vi "Translator.vi"(0 "Input":variant, 11 "error in (no error)":errorcluster) -> (4 "Output":variant, 15 "error out":errorcluster)   [LabVIEW 2014, in "Complex Numbers.lvlib"]
doc: "An example of how to create the Translator to convert the LabVIEW VIs to Arduino C code."
uses:
  Complex Numbers.lvlib
panel:
  out "Outputs":string[](array[string])
  out "Inputs":string[](array[string])
  out "Output Datatypes":string[](array[string])
  out "Input Datatypes":string[](array[string])
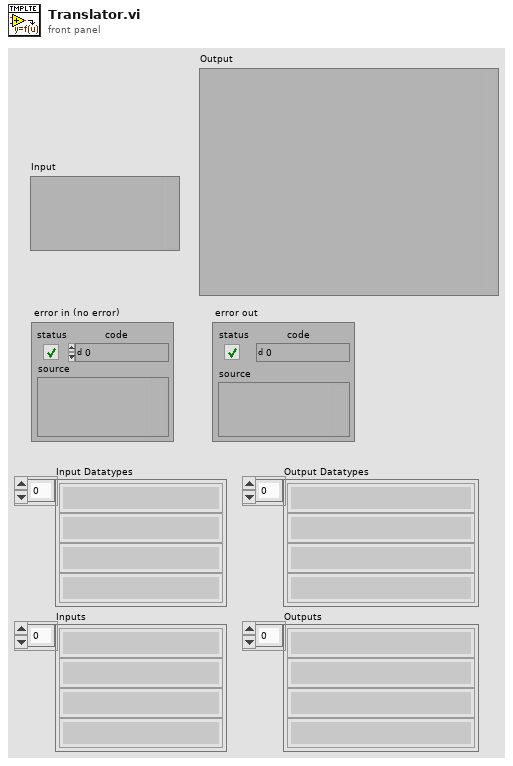
[diagram p1: front panel]
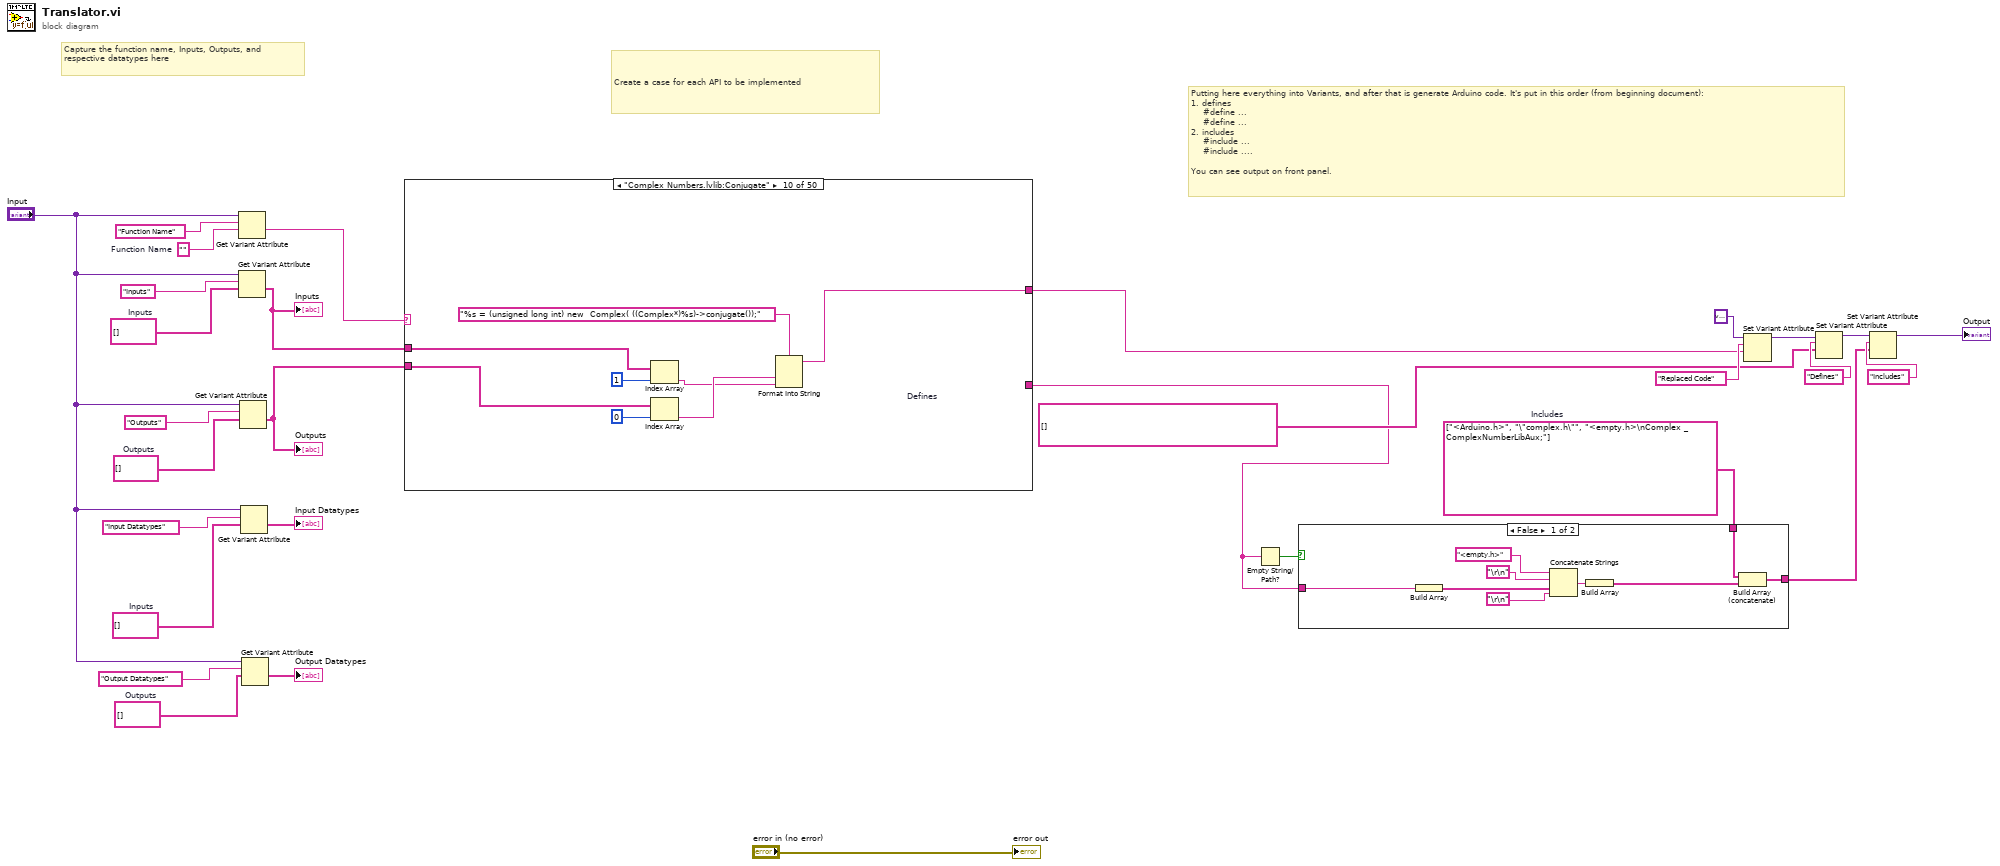
[diagram p0: block diagram]
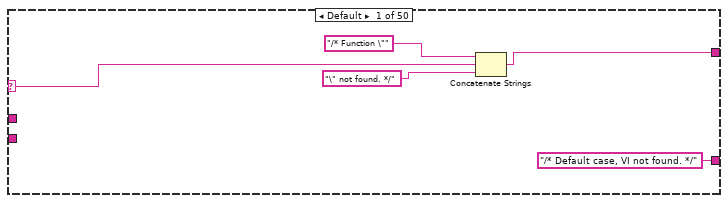
[diagram p3: hidden frame]
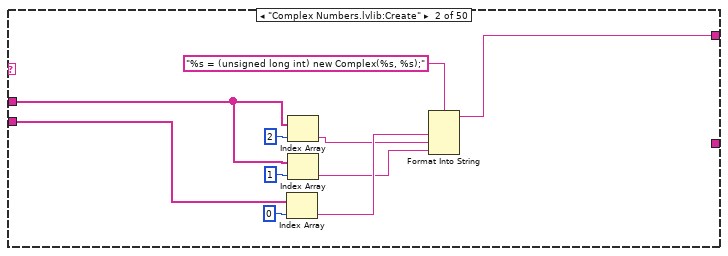
[diagram p4: hidden frame]
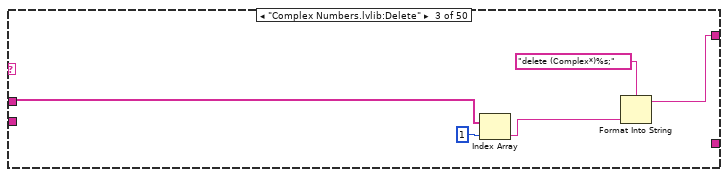
[diagram p5: hidden frame]
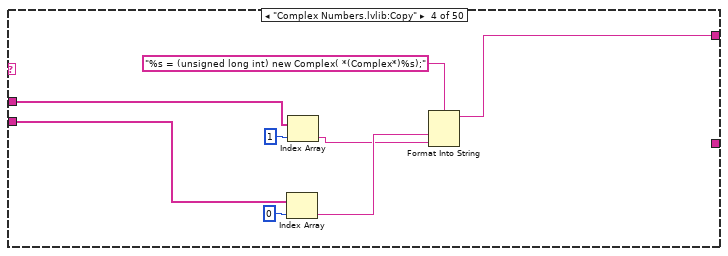
[diagram p6: hidden frame]
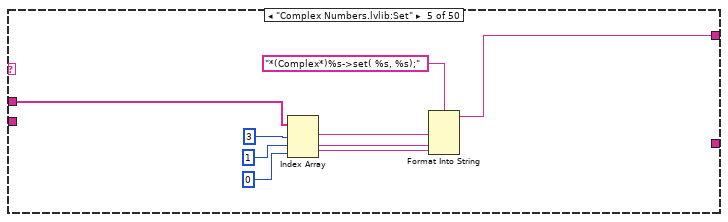
[diagram p7: hidden frame]
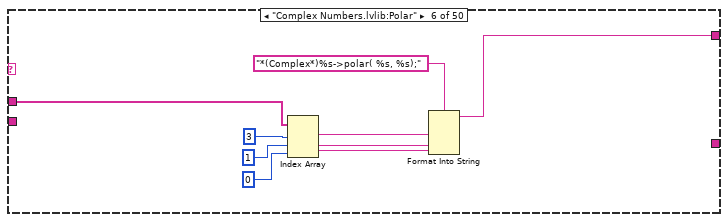
[diagram p8: hidden frame]
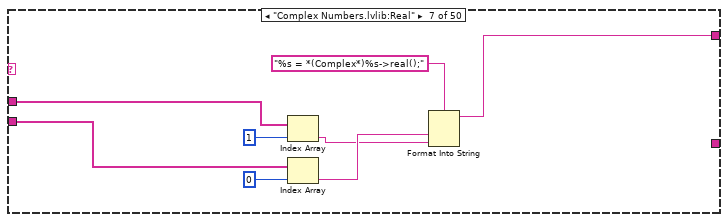
[diagram p9: hidden frame]
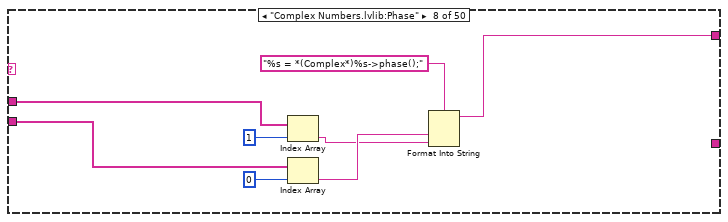
[diagram p10: hidden frame]
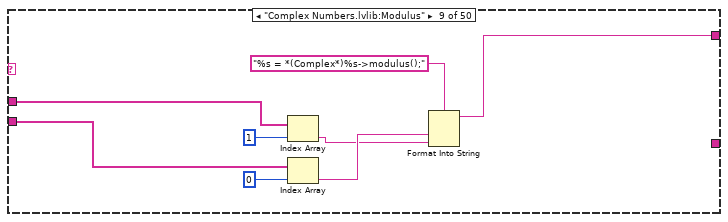
[diagram p11: hidden frame]
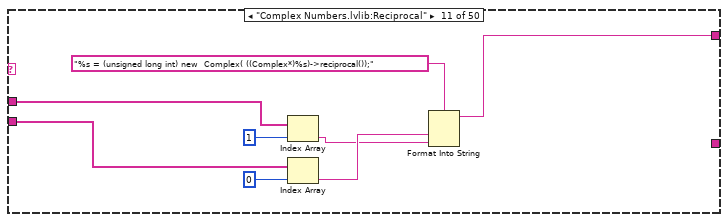
[diagram p12: hidden frame]
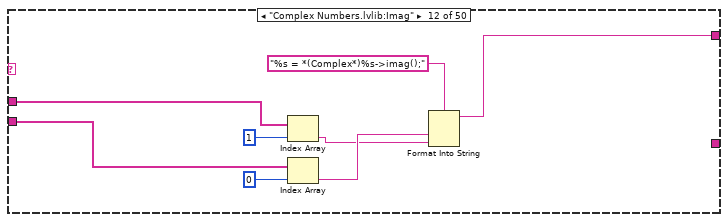
[diagram p13: hidden frame]
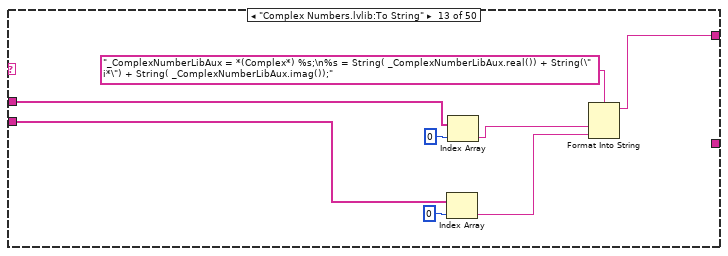
[diagram p14: hidden frame]
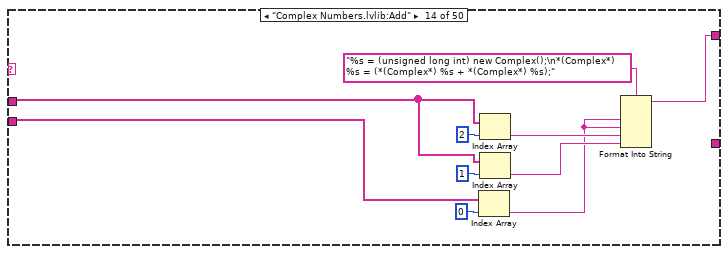
[diagram p15: hidden frame]
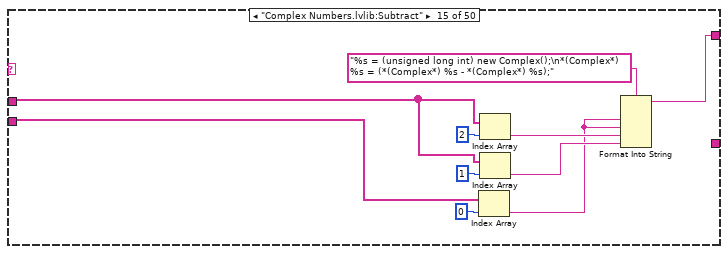
[diagram p16: hidden frame]
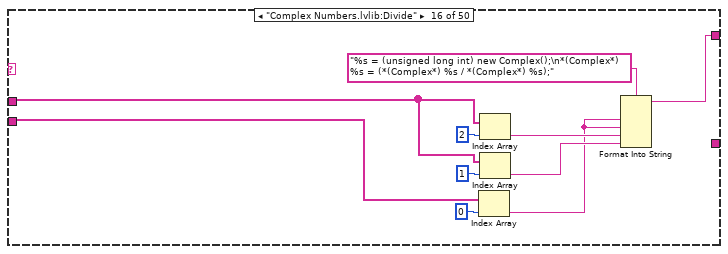
[diagram p17: hidden frame]
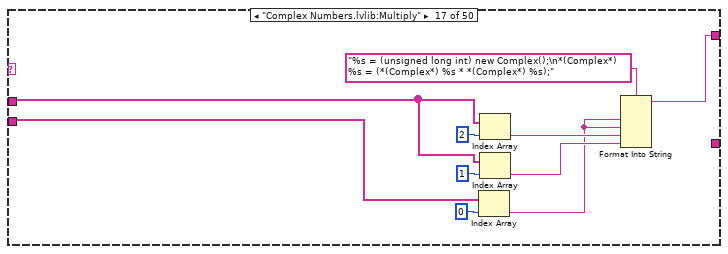
[diagram p18: hidden frame]
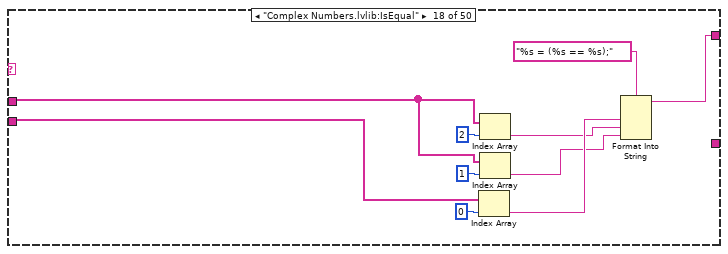
[diagram p19: hidden frame]
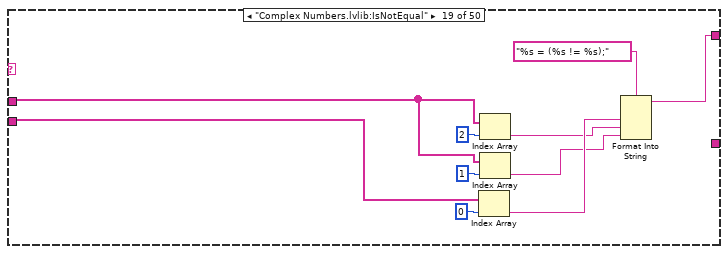
[diagram p20: hidden frame]
diagram:
  w4 = string[] []  # Defines
  w19 = string[] []  # Outputs
  w20 = string[] []  # Inputs
  w1 = string[] ["<Arduino.h>", "\"complex.h\"", "<empty.h>\nComplex _ComplexNumberLibAux;"]  # Includes
  w26 = string[] []  # Outputs
  w27 = string[] []  # Inputs
  w28 = ""  # Function Name
  # "Capture the function name, Inputs, Outputs, and respective datatypes here"
  # "Putting here everything into Variants, and after that is generate Arduino code. It's put in this order (from beginning document):\n1. defines\n    #define ...\n    #define ...\n2. includes\n    #include ...\n    #include ....\n\nYou can see output on front panel."
  # "Create a case for each API to be implemented"
  n1 = Get Variant Attribute(Variant="Input", name="Function Name", default value (empty Variant)=w28) -> (value=w10:string)  [unwired: 1 in, 3 out]
  n2 = Get Variant Attribute(Variant="Input", name="Inputs", default value (empty Variant)=w27) -> (value=w9:string[])  [unwired: 1 in, 3 out]
  "Inputs" <- w9
  n3 = Get Variant Attribute(Variant="Input", name="Outputs", default value (empty Variant)=w26) -> (value=w8:string[])  [unwired: 1 in, 3 out]
  "Outputs" <- w8
  n4 = Get Variant Attribute(Variant="Input", name="Input Datatypes", default value (empty Variant)=w20) -> (value=→"Input Datatypes":string[])  [unwired: 1 in, 3 out]
  n5 = Get Variant Attribute(Variant="Input", name="Output Datatypes", default value (empty Variant)=w19) -> (value=→"Output Datatypes":string[])  [unwired: 1 in, 3 out]
  n6 = case shown="\"Complex Numbers.lvlib:Conjugate\"" w10 {
    selector: w10 -> [w33 _ _ _ _ _ _ _ _ _ _ _ _ _ _ _ _ _ _ _ _ _ _ _ _ _ _ _ _ _ _ _ _ _ _ _ _ _ _ _ _ _ _ _ _ _ _ _ _ _]
    tunnel: w9 -> [_ w38 w48 w52 w64 w73 w80 w88 w96 w104 w112 w120 w126 w136 w146 w156 w166 w177 w187 w196 w204 w210 w222 w230 w238 w244 w256 w264 w272 w280 w288 w296 w304 w312 w320 w328 w336 w344 w352 w360 w368 w376 w384 w392 w400 w408 w416 w424 w432 w440]
    tunnel: w8 -> [_ w42 _ w55 _ _ w79 w87 w95 w103 w111 w119 w129 w138 w148 w158 w168 w179 w189 w197 w205 w215 w223 w231 w239 w249 w257 w265 w273 w281 w289 w297 w305 w313 w321 w329 w337 w345 w353 w361 w369 w377 w385 w393 w401 w409 w417 w425 w433 w441]
    tunnel: [w31 w41 w47 w54 w66 w75 w83 w91 w99 w107 w115 w123 w128 w134 w144 w154 w164 w176 w186 w195 w203 w214 w221 w229 w237 w248 w255 w263 w271 w279 w287 w295 w303 w311 w319 w327 w335 w343 w351 w359 w367 w375 w383 w391 w399 w407 w415 w423 w431 w439] -> w7
    tunnel: ["/* Default case, VI not found. */" ("name") _ _ _ _ _ _ _ _ _ _ _ _ _ _ _ _ _ _ _ _ _ _ _ _ _ _ _ _ _ _ _ _ _ _ _ _ _ _ _ _ _ _ _ _ _ _ _ _ _] -> w3
    frame Default {
      n7 = Concatenate Strings("/* Function \"" ("string"), w33, "\" not found. */" ("string")) -> (w31:string)
    }
    frame "Complex Numbers.lvlib:Create" {
      n8 = Index Array(array=w42, index=0) -> (element=w44:string)
      n9 = Index Array(array=w38, index=2) -> (element=w37:string)
      n10 = Index Array(array=w38, index=1) -> (element=w36:string)
      n11 = Format Into String(format string="%s = (unsigned long int) new Complex(%s, %s);", w44, w37, w36) -> (resulting string=w41:string)  [unwired: 2 in, 1 out]
    }
    frame "Complex Numbers.lvlib:Delete" {
      n12 = Index Array(array=w48, index=1) -> (element=w46:string)
      n13 = Format Into String(format string="delete (Complex*)%s;", w46) -> (resulting string=w47:string)  [unwired: 2 in, 1 out]
    }
    frame "Complex Numbers.lvlib:Copy" {
      n14 = Index Array(array=w55, index=0) -> (element=w57:string)
      n15 = Index Array(array=w52, index=1) -> (element=w51:string)
      n16 = Format Into String(format string="%s = (unsigned long int) new Complex( *(Complex*)%s);", w57, w51) -> (resulting string=w54:string)  [unwired: 2 in, 1 out]
    }
    frame "Complex Numbers.lvlib:Set" {
      n17 = Index Array(array=w64, index #1=3 ("index"), index #2=1 ("index"), index #3=0 ("index")) -> (element #1=w61:string, element #2=w60:string, element #3=w59:string)
      n18 = Format Into String(format string="*(Complex*)%s->set( %s, %s);", w61, w60, w59) -> (resulting string=w66:string)  [unwired: 2 in, 1 out]
    }
    frame "Complex Numbers.lvlib:Polar" {
      n19 = Index Array(array=w73, index #1=3 ("index"), index #2=1 ("index"), index #3=0 ("index")) -> (element #1=w70:string, element #2=w69:string, element #3=w68:string)
      n20 = Format Into String(format string="*(Complex*)%s->polar( %s, %s);", w70, w69, w68) -> (resulting string=w75:string)  [unwired: 2 in, 1 out]
    }
    frame "Complex Numbers.lvlib:Real" {
      n21 = Index Array(array=w80, index=1) -> (element=w77:string)
      n22 = Index Array(array=w79, index=0) -> (element=w78:string)
      n23 = Format Into String(format string="%s = *(Complex*)%s->real();", w78, w77) -> (resulting string=w83:string)  [unwired: 2 in, 1 out]
    }
    frame "Complex Numbers.lvlib:Phase" {
      n24 = Index Array(array=w88, index=1) -> (element=w85:string)
      n25 = Index Array(array=w87, index=0) -> (element=w86:string)
      n26 = Format Into String(format string="%s = *(Complex*)%s->phase();", w86, w85) -> (resulting string=w91:string)  [unwired: 2 in, 1 out]
    }
    frame "Complex Numbers.lvlib:Modulus" {
      n27 = Index Array(array=w96, index=1) -> (element=w93:string)
      n28 = Index Array(array=w95, index=0) -> (element=w94:string)
      n29 = Format Into String(format string="%s = *(Complex*)%s->modulus();", w94, w93) -> (resulting string=w99:string)  [unwired: 2 in, 1 out]
    }
    frame "Complex Numbers.lvlib:Conjugate" {
      n30 = Index Array(array=w104, index=1) -> (element=w101:string)
      n31 = Index Array(array=w103, index=0) -> (element=w102:string)
      n32 = Format Into String(format string="%s = (unsigned long int) new  Complex( ((Complex*)%s)->conjugate());", w102, w101) -> (resulting string=w107:string)  [unwired: 2 in, 1 out]
    }
    frame "Complex Numbers.lvlib:Reciprocal" {
      n33 = Index Array(array=w112, index=1) -> (element=w109:string)
      n34 = Index Array(array=w111, index=0) -> (element=w110:string)
      n35 = Format Into String(format string="%s = (unsigned long int) new  Complex( ((Complex*)%s)->reciprocal());", w110, w109) -> (resulting string=w115:string)  [unwired: 2 in, 1 out]
    }
    frame "Complex Numbers.lvlib:Imag" {
      n36 = Index Array(array=w120, index=1) -> (element=w117:string)
      n37 = Index Array(array=w119, index=0) -> (element=w118:string)
      n38 = Format Into String(format string="%s = *(Complex*)%s->imag();", w118, w117) -> (resulting string=w123:string)  [unwired: 2 in, 1 out]
    }
    frame "Complex Numbers.lvlib:To String" {
      n39 = Index Array(array=w129, index=0) -> (element=w131:string)
      n40 = Index Array(array=w126, index=0) -> (element=w125:string)
      n41 = Format Into String(format string="_ComplexNumberLibAux = *(Complex*) %s;\n%s = String( _ComplexNumberLibAux.real()) + String(\" i*\") + String( _ComplexNumberLibAux.imag());", w125, w131) -> (resulting string=w128:string)  [unwired: 2 in, 1 out]
    }
    frame "Complex Numbers.lvlib:Add" {
      n42 = Index Array(array=w138, index=0) -> (element=w133:string)
      n43 = Index Array(array=w136, index=2) -> (element=w142:string)
      n44 = Index Array(array=w136, index=1) -> (element=w135:string)
      n45 = Format Into String(format string="%s = (unsigned long int) new Complex();\n*(Complex*) %s = (*(Complex*) %s + *(Complex*) %s);", w133, w133, w142, w135) -> (resulting string=w134:string)  [unwired: 2 in, 1 out]
    }
    frame "Complex Numbers.lvlib:Subtract" {
      n46 = Index Array(array=w148, index=0) -> (element=w143:string)
      n47 = Index Array(array=w146, index=2) -> (element=w152:string)
      n48 = Index Array(array=w146, index=1) -> (element=w145:string)
      n49 = Format Into String(format string="%s = (unsigned long int) new Complex();\n*(Complex*) %s = (*(Complex*) %s - *(Complex*) %s);", w143, w143, w152, w145) -> (resulting string=w144:string)  [unwired: 2 in, 1 out]
    }
    frame "Complex Numbers.lvlib:Divide" {
      n50 = Index Array(array=w158, index=0) -> (element=w153:string)
      n51 = Index Array(array=w156, index=2) -> (element=w162:string)
      n52 = Index Array(array=w156, index=1) -> (element=w155:string)
      n53 = Format Into String(format string="%s = (unsigned long int) new Complex();\n*(Complex*) %s = (*(Complex*) %s / *(Complex*) %s);", w153, w153, w162, w155) -> (resulting string=w154:string)  [unwired: 2 in, 1 out]
    }
    frame "Complex Numbers.lvlib:Multiply" {
      n54 = Index Array(array=w168, index=0) -> (element=w163:string)
      n55 = Index Array(array=w166, index=2) -> (element=w172:string)
      n56 = Index Array(array=w166, index=1) -> (element=w165:string)
      n57 = Format Into String(format string="%s = (unsigned long int) new Complex();\n*(Complex*) %s = (*(Complex*) %s * *(Complex*) %s);", w163, w163, w172, w165) -> (resulting string=w164:string)  [unwired: 2 in, 1 out]
    }
    frame "Complex Numbers.lvlib:IsEqual" {
      n58 = Index Array(array=w179, index=0) -> (element=w175:string)
      n59 = Index Array(array=w177, index=2) -> (element=w174:string)
      n60 = Index Array(array=w177, index=1) -> (element=w173:string)
      n61 = Format Into String(format string="%s = (%s == %s);", w175, w174, w173) -> (resulting string=w176:string)  [unwired: 2 in, 1 out]
    }
    frame "Complex Numbers.lvlib:IsNotEqual" {
      n62 = Index Array(array=w189, index=0) -> (element=w185:string)
      n63 = Index Array(array=w187, index=2) -> (element=w184:string)
      n64 = Index Array(array=w187, index=1) -> (element=w183:string)
      n65 = Format Into String(format string="%s = (%s != %s);", w185, w184, w183) -> (resulting string=w186:string)  [unwired: 2 in, 1 out]
    }
    frame "Complex Numbers.lvlib:Sqr" {
      n66 = Index Array(array=w197, index=0) -> (element=w194:string)
      n67 = Index Array(array=w196, index=1) -> (element=w193:string)
      n68 = Format Into String(format string="%s = (unsigned long int) new Complex( ((Complex*)%s)->c_sqr());", w194, w193) -> (resulting string=w195:string)  [unwired: 2 in, 1 out]
    }
    frame "Complex Numbers.lvlib:Sqrt" {
      n69 = Index Array(array=w205, index=0) -> (element=w202:string)
      n70 = Index Array(array=w204, index=1) -> (element=w201:string)
      n71 = Format Into String(format string="%s = (unsigned long int) new Complex( ((Complex*)%s)->c_sqrt());", w202, w201) -> (resulting string=w203:string)  [unwired: 2 in, 1 out]
    }
    frame "Complex Numbers.lvlib:Pow" {
      n72 = Index Array(array=w215, index=0) -> (element=w213:string)
      n73 = Index Array(array=w210, index=2) -> (element=w212:string)
      n74 = Index Array(array=w210, index=1) -> (element=w209:string)
      n75 = Format Into String(format string="%s = (unsigned long int) new Complex( ((Complex*)%s)->c_pow( *(Complex*)%s));", w213, w212, w209) -> (resulting string=w214:string)  [unwired: 2 in, 1 out]
    }
    frame "Complex Numbers.lvlib:Exp" {
      n76 = Index Array(array=w223, index=0) -> (element=w220:string)
      n77 = Index Array(array=w222, index=1) -> (element=w219:string)
      n78 = Format Into String(format string="%s = (unsigned long int) new Complex( ((Complex*)%s)->c_exp());", w220, w219) -> (resulting string=w221:string)  [unwired: 2 in, 1 out]
    }
    frame "Complex Numbers.lvlib:Log" {
      n79 = Index Array(array=w231, index=0) -> (element=w228:string)
      n80 = Index Array(array=w230, index=1) -> (element=w227:string)
      n81 = Format Into String(format string="%s = (unsigned long int) new Complex( ((Complex*)%s)->c_log());", w228, w227) -> (resulting string=w229:string)  [unwired: 2 in, 1 out]
    }
    frame "Complex Numbers.lvlib:Log10" {
      n82 = Index Array(array=w239, index=0) -> (element=w236:string)
      n83 = Index Array(array=w238, index=1) -> (element=w235:string)
      n84 = Format Into String(format string="%s = (unsigned long int) new Complex( ((Complex*)%s)->c_log10());", w236, w235) -> (resulting string=w237:string)  [unwired: 2 in, 1 out]
    }
    frame "Complex Numbers.lvlib:LogN" {
      n85 = Index Array(array=w249, index=0) -> (element=w247:string)
      n86 = Index Array(array=w244, index=2) -> (element=w246:string)
      n87 = Index Array(array=w244, index=1) -> (element=w243:string)
      n88 = Format Into String(format string="%s = (unsigned long int) new Complex( ((Complex*)%s)->c_logn( *(Complex*)%s));", w247, w246, w243) -> (resulting string=w248:string)  [unwired: 2 in, 1 out]
    }
    frame "Complex Numbers.lvlib:Sin" {
      n89 = Index Array(array=w257, index=0) -> (element=w254:string)
      n90 = Index Array(array=w256, index=1) -> (element=w253:string)
      n91 = Format Into String(format string="%s = (unsigned long int) new Complex( ((Complex*)%s)->c_sin());", w254, w253) -> (resulting string=w255:string)  [unwired: 2 in, 1 out]
    }
    frame "Complex Numbers.lvlib:Cos" {
      n92 = Index Array(array=w265, index=0) -> (element=w262:string)
      n93 = Index Array(array=w264, index=1) -> (element=w261:string)
      n94 = Format Into String(format string="%s = (unsigned long int) new Complex( ((Complex*)%s)->c_cos());", w262, w261) -> (resulting string=w263:string)  [unwired: 2 in, 1 out]
    }
    frame "Complex Numbers.lvlib:Tan" {
      n95 = Index Array(array=w273, index=0) -> (element=w270:string)
      n96 = Index Array(array=w272, index=1) -> (element=w269:string)
      n97 = Format Into String(format string="%s = (unsigned long int) new Complex( ((Complex*)%s)->c_tan());", w270, w269) -> (resulting string=w271:string)  [unwired: 2 in, 1 out]
    }
    frame "Complex Numbers.lvlib:Cot" {
      n98 = Index Array(array=w281, index=0) -> (element=w278:string)
      n99 = Index Array(array=w280, index=1) -> (element=w277:string)
      n100 = Format Into String(format string="%s = (unsigned long int) new Complex( ((Complex*)%s)->c_cot());", w278, w277) -> (resulting string=w279:string)  [unwired: 2 in, 1 out]
    }
    frame "Complex Numbers.lvlib:Asin" {
      n101 = Index Array(array=w289, index=0) -> (element=w286:string)
      n102 = Index Array(array=w288, index=1) -> (element=w285:string)
      n103 = Format Into String(format string="%s = (unsigned long int) new Complex( ((Complex*)%s)->c_asin());", w286, w285) -> (resulting string=w287:string)  [unwired: 2 in, 1 out]
    }
    frame "Complex Numbers.lvlib:Acos" {
      n104 = Index Array(array=w297, index=0) -> (element=w294:string)
      n105 = Index Array(array=w296, index=1) -> (element=w293:string)
      n106 = Format Into String(format string="%s = (unsigned long int) new Complex( ((Complex*)%s)->c_acos());", w294, w293) -> (resulting string=w295:string)  [unwired: 2 in, 1 out]
    }
    frame "Complex Numbers.lvlib:Atan" {
      n107 = Index Array(array=w305, index=0) -> (element=w302:string)
      n108 = Index Array(array=w304, index=1) -> (element=w301:string)
      n109 = Format Into String(format string="%s = (unsigned long int) new Complex( ((Complex*)%s)->c_atan());", w302, w301) -> (resulting string=w303:string)  [unwired: 2 in, 1 out]
    }
    frame "Complex Numbers.lvlib:Acot" {
      n110 = Index Array(array=w313, index=0) -> (element=w310:string)
      n111 = Index Array(array=w312, index=1) -> (element=w309:string)
      n112 = Format Into String(format string="%s = (unsigned long int) new Complex( ((Complex*)%s)->c_acot());", w310, w309) -> (resulting string=w311:string)  [unwired: 2 in, 1 out]
    }
    frame "Complex Numbers.lvlib:Csc" {
      n113 = Index Array(array=w321, index=0) -> (element=w318:string)
      n114 = Index Array(array=w320, index=1) -> (element=w317:string)
      n115 = Format Into String(format string="%s = (unsigned long int) new Complex( ((Complex*)%s)->c_csc());", w318, w317) -> (resulting string=w319:string)  [unwired: 2 in, 1 out]
    }
    frame "Complex Numbers.lvlib:Sec" {
      n116 = Index Array(array=w329, index=0) -> (element=w326:string)
      n117 = Index Array(array=w328, index=1) -> (element=w325:string)
      n118 = Format Into String(format string="%s = (unsigned long int) new Complex( ((Complex*)%s)->c_sec());", w326, w325) -> (resulting string=w327:string)  [unwired: 2 in, 1 out]
    }
    frame "Complex Numbers.lvlib:Acsc" {
      n119 = Index Array(array=w337, index=0) -> (element=w334:string)
      n120 = Index Array(array=w336, index=1) -> (element=w333:string)
      n121 = Format Into String(format string="%s = (unsigned long int) new Complex( ((Complex*)%s)->c_acsc());", w334, w333) -> (resulting string=w335:string)  [unwired: 2 in, 1 out]
    }
    frame "Complex Numbers.lvlib:Asec" {
      n122 = Index Array(array=w345, index=0) -> (element=w342:string)
      n123 = Index Array(array=w344, index=1) -> (element=w341:string)
      n124 = Format Into String(format string="%s = (unsigned long int) new Complex( ((Complex*)%s)->c_asec());", w342, w341) -> (resulting string=w343:string)  [unwired: 2 in, 1 out]
    }
    frame "Complex Numbers.lvlib:Sinh" {
      n125 = Index Array(array=w353, index=0) -> (element=w350:string)
      n126 = Index Array(array=w352, index=1) -> (element=w349:string)
      n127 = Format Into String(format string="%s = (unsigned long int) new Complex( ((Complex*)%s)->c_sinh());", w350, w349) -> (resulting string=w351:string)  [unwired: 2 in, 1 out]
    }
    frame "Complex Numbers.lvlib:Cosh" {
      n128 = Index Array(array=w361, index=0) -> (element=w358:string)
      n129 = Index Array(array=w360, index=1) -> (element=w357:string)
      n130 = Format Into String(format string="%s = (unsigned long int) new Complex( ((Complex*)%s)->c_cosh());", w358, w357) -> (resulting string=w359:string)  [unwired: 2 in, 1 out]
    }
    frame "Complex Numbers.lvlib:Tanh" {
      n131 = Index Array(array=w369, index=0) -> (element=w366:string)
      n132 = Index Array(array=w368, index=1) -> (element=w365:string)
      n133 = Format Into String(format string="%s = (unsigned long int) new Complex( ((Complex*)%s)->c_tanh());", w366, w365) -> (resulting string=w367:string)  [unwired: 2 in, 1 out]
    }
    frame "Complex Numbers.lvlib:Asinh" {
      n134 = Index Array(array=w377, index=0) -> (element=w374:string)
      n135 = Index Array(array=w376, index=1) -> (element=w373:string)
      n136 = Format Into String(format string="%s = (unsigned long int) new Complex( ((Complex*)%s)->c_asinh());", w374, w373) -> (resulting string=w375:string)  [unwired: 2 in, 1 out]
    }
    frame "Complex Numbers.lvlib:Acosh" {
      n137 = Index Array(array=w385, index=0) -> (element=w382:string)
      n138 = Index Array(array=w384, index=1) -> (element=w381:string)
      n139 = Format Into String(format string="%s = (unsigned long int) new Complex( ((Complex*)%s)->c_acosh());", w382, w381) -> (resulting string=w383:string)  [unwired: 2 in, 1 out]
    }
    frame "Complex Numbers.lvlib:Atanh" {
      n140 = Index Array(array=w393, index=0) -> (element=w390:string)
      n141 = Index Array(array=w392, index=1) -> (element=w389:string)
      n142 = Format Into String(format string="%s = (unsigned long int) new Complex( ((Complex*)%s)->c_atanh());", w390, w389) -> (resulting string=w391:string)  [unwired: 2 in, 1 out]
    }
    frame "Complex Numbers.lvlib:Sech" {
      n143 = Index Array(array=w401, index=0) -> (element=w398:string)
      n144 = Index Array(array=w400, index=1) -> (element=w397:string)
      n145 = Format Into String(format string="%s = (unsigned long int) new Complex( ((Complex*)%s)->c_sech());", w398, w397) -> (resulting string=w399:string)  [unwired: 2 in, 1 out]
    }
    frame "Complex Numbers.lvlib:Csch" {
      n146 = Index Array(array=w409, index=0) -> (element=w406:string)
      n147 = Index Array(array=w408, index=1) -> (element=w405:string)
      n148 = Format Into String(format string="%s = (unsigned long int) new Complex( ((Complex*)%s)->c_csch());", w406, w405) -> (resulting string=w407:string)  [unwired: 2 in, 1 out]
    }
    frame "Complex Numbers.lvlib:Coth" {
      n149 = Index Array(array=w417, index=0) -> (element=w414:string)
      n150 = Index Array(array=w416, index=1) -> (element=w413:string)
      n151 = Format Into String(format string="%s = (unsigned long int) new Complex( ((Complex*)%s)->c_coth());", w414, w413) -> (resulting string=w415:string)  [unwired: 2 in, 1 out]
    }
    frame "Complex Numbers.lvlib:Asech" {
      n152 = Index Array(array=w425, index=0) -> (element=w422:string)
      n153 = Index Array(array=w424, index=1) -> (element=w421:string)
      n154 = Format Into String(format string="%s = (unsigned long int) new Complex( ((Complex*)%s)->c_asech());", w422, w421) -> (resulting string=w423:string)  [unwired: 2 in, 1 out]
    }
    frame "Complex Numbers.lvlib:Acsch" {
      n155 = Index Array(array=w433, index=0) -> (element=w430:string)
      n156 = Index Array(array=w432, index=1) -> (element=w429:string)
      n157 = Format Into String(format string="%s = (unsigned long int) new Complex( ((Complex*)%s)->c_acsch());", w430, w429) -> (resulting string=w431:string)  [unwired: 2 in, 1 out]
    }
    frame "Complex Numbers.lvlib:Acoth" {
      n158 = Index Array(array=w441, index=0) -> (element=w438:string)
      n159 = Index Array(array=w440, index=1) -> (element=w437:string)
      n160 = Format Into String(format string="%s = (unsigned long int) new Complex( ((Complex*)%s)->c_acoth());", w438, w437) -> (resulting string=w439:string)  [unwired: 2 in, 1 out]
    }
  }
  n161 = Empty String/Path?(string/path=w3) -> (empty?=w5:bool)
  n162 = case shown="False" w5 {
    tunnel: w3 -> [w453 _]
    tunnel: [w446 w454] -> w2
    tunnel: w1 -> [w445 w454]
    frame False {
      n163 = Build Array(w453) -> (w447:string[])
      n164 = Concatenate Strings("<empty.h>" ("string"), "\r\n", w447, "\r\n") -> (w448:string)
      n165 = Build Array(w448) -> (w452:string[])
      n166 = Build Array (concatenate)(w445, w452) -> (w446:string[])
    }
    frame True {
    }
  }
  n167 = Set Variant Attribute(Variant=variant ("variant"), name="Replaced Code", value=w7) -> (Variant out=w13:variant)  [unwired: 1 in, 2 out]
  n168 = Set Variant Attribute(Variant=w13, name="Defines", value=w4) -> (Variant out=w12:variant)  [unwired: 1 in, 2 out]
  n169 = Set Variant Attribute(Variant=w12, name="Includes", value=w2) -> (Variant out=→"Output":variant)  [unwired: 1 in, 2 out]
  "error out" <- "error in (no error)"
